vi "Update lvcsm Section in VI Description.vi"(8 "error in (no error)":errorcluster, 11 "CSM-Helper in":refnum<class "CSM-Helper.lvclass">) -> (0 "error out":errorcluster, 3 "CSM-Helper out":refnum<class "CSM-Helper.lvclass">)   [LabVIEW 2017, in "CSM-Helper.lvclass"]
uses:
  CSM-Helper.lvclass
  CSM-Helper.lvclass/CSM-Helper.ctl
  _Shared/Trim Single-line Text.vi
  _Shared/CSM Shared.lvlib
  Communicable State Machine.lvlib
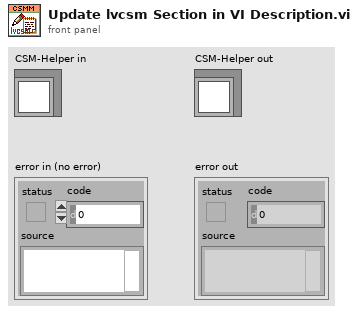
[diagram p1: front panel]
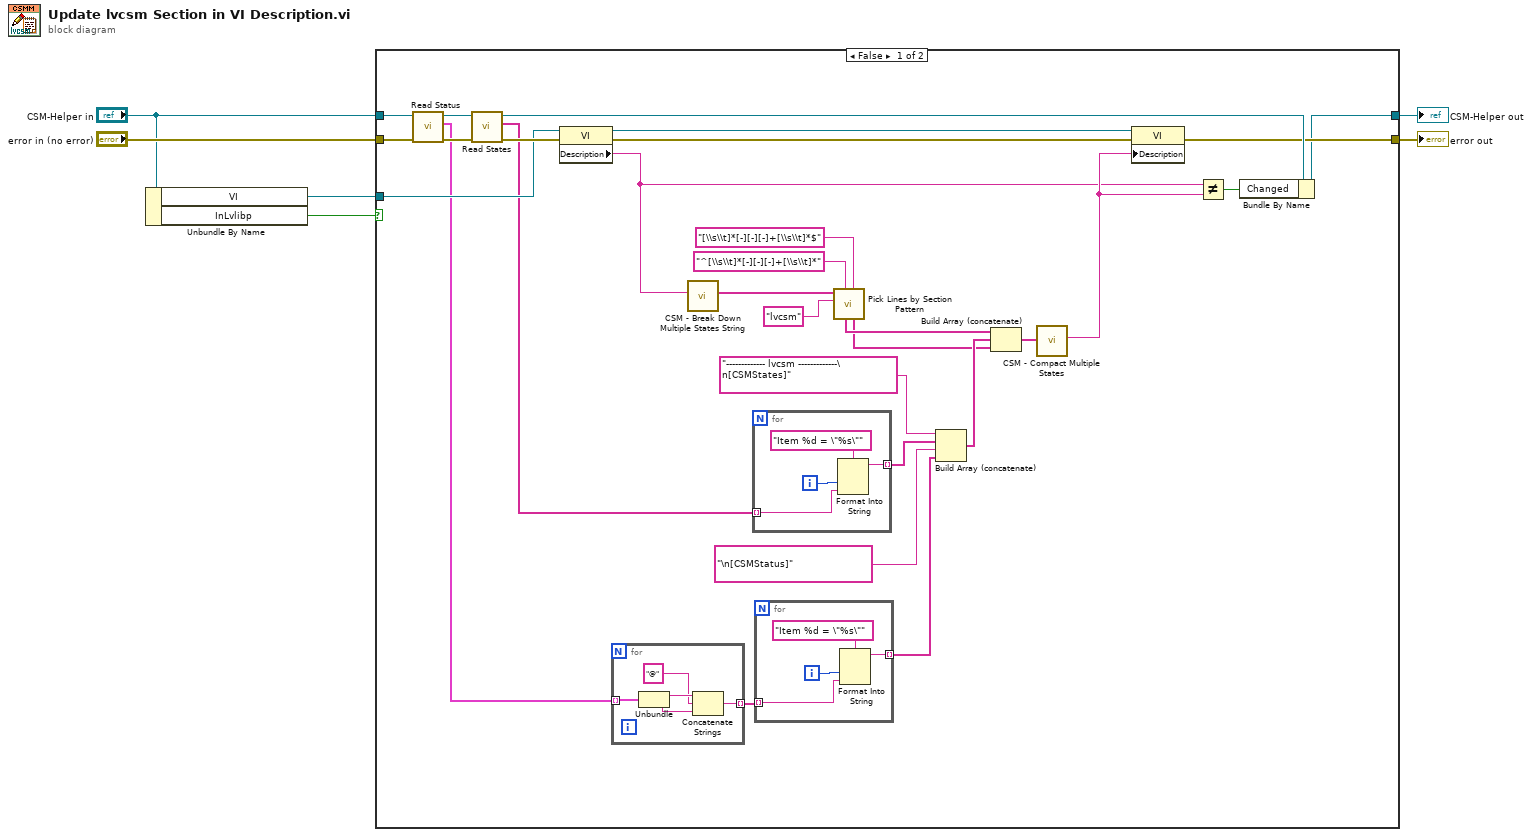
[diagram p0: block diagram]
diagram:
  n1 = Unbundle By Name("CSM-Helper in") -> ("VI"=w2:refnum<vi>, "InLvlibp"=w1:bool)
  n2 = case shown="False" w1 {
    tunnel: "error in (no error)" -> [w14 w49]
    tunnel: [w20 w49] -> w5
    tunnel: [w18 w50] -> w4
    tunnel: "CSM-Helper in" -> [w11 w50]
    tunnel: w2 -> [w33 _]
    frame False {
      n3 = call "Read Status.vi"("error in (no error)"=w14, "CSM-Helper in"=w11) -> ("error out"=w13:errorcluster, "Array 3"=w10:cluster{"Status":string, "InState":string}[], "CSM-Helper out"=w12:refnum<class "CSM-Helper.lvclass">)  [unwired: 7 in]
      n4 = call "Read States.vi"("error in (no error)"=w13, "CSM-Helper in"=w12) -> ("error out"=w34:errorcluster, "Value"=w28:string[], "CSM-Helper out"=w35:refnum<class "CSM-Helper.lvclass">)  [unwired: 7 in]
      n5 = property class="VI"(reference=w33, error in=w34) -> (reference out=w19:refnum<vi>, error out=w21:errorcluster, "Description"=w15:string)
      n6 = for {
        tunnel: w10 -> [w44] mode=indexing
        tunnel: [w40] -> w9 mode=indexing
        n7 = Unbundle(w44) -> ("Status"=w43:string, "InState"=w42:string)
        n8 = Concatenate Strings(w43, "@" ("string"), w42) -> (w40:string)
      }
      n9 = call "CSM - Break Down Multiple States String.vi"("States"=w15) -> ("Multiple States"=w29:string[])  [unwired: 10 in]
      n10 = for {
        tunnel: w28 -> [w47] mode=indexing
        tunnel: [w45] -> w27 mode=indexing
        i -> [w46]
        n11 = Format Into String(format string="Item %d = \"%s\"", w46, w47) -> (resulting string=w45:string)  [unwired: 2 in, 1 out]
      }
      n12 = for {
        tunnel: w9 -> [w38] mode=indexing
        tunnel: [w36] -> w7 mode=indexing
        i -> [w37]
        n13 = Format Into String(format string="Item %d = \"%s\"", w37, w38) -> (resulting string=w36:string)  [unwired: 2 in, 1 out]
      }
      n14 = call "Pick Lines by Section Pattern.vi"("RegExp Right(\"^[\")"="[\\s\\t]*[-][-][-]+[\\s\\t]*$" ("RegExp Lef(\"^[\")"), "RegExp Lef(\"^[\")"="^[\\s\\t]*[-][-][-]+[\\s\\t]*" ("RegExp Lef(\"^[\")"), "Session Name"="lvcsm" ("[] Session Name"), "Config Text List"=w29) -> ("End"=w23:string[], "Front"=w24:string[])  [unwired: 3 in, 3 out]
      n15 = Build Array (concatenate)("------------- lvcsm -------------\n[CSMStates]" ("RegExp Lef(\"^[\")"), w27, "\n[CSMStatus]" ("RegExp Lef(\"^[\")"), w7) -> (w25:string[])
      n16 = Build Array (concatenate)(w24, w25, w23) -> (w22:string[])
      n17 = call "CSM - Compact Multiple States.vi"("Multiple States"=w22) -> ("States"=w16:string)  [unwired: 9 in]
      n18 = property class="VI"(reference=w19, error in=w21, "Description"=w16) -> (error out=w20:errorcluster)  [unwired: 1 out]
      n19 = Not Equal?(x=w15, y=w16) -> (x != y?=w17:bool)
      n20 = Bundle By Name(cluster=w35, "Changed"=w17) -> (w18:refnum<class "CSM-Helper.lvclass">)
    }
    frame True {
    }
  }
  "error out" <- w5
  "CSM-Helper out" <- w4
